vi "ParseAgentMessageChunk.vi"(8 "Error In":errorcluster, 9 "AgentMessage":T5, 10 "SessionId":string, 11 "LiteAgent In":T1) -> (0 "Error Out":errorcluster, 1 "Completions":T3, 2 "Part":T2, 3 "LiteAgent Out":T1, 5 "Common":T4)   [LabVIEW 2017]
uses:
  C:/Users/Jan/Projects/LiteAgentSDK-LabVIEW/Source/Bin/LiteAgentSDK.LabVIEW.dll
  Bin/LiteAgentSDK.LabVIEW.dll
  <vilib>/LVH/i3 JSON/i3-json.lvlib
  <vilib>/addons/Tools/Unicode/UTF8 Tools.lvlib
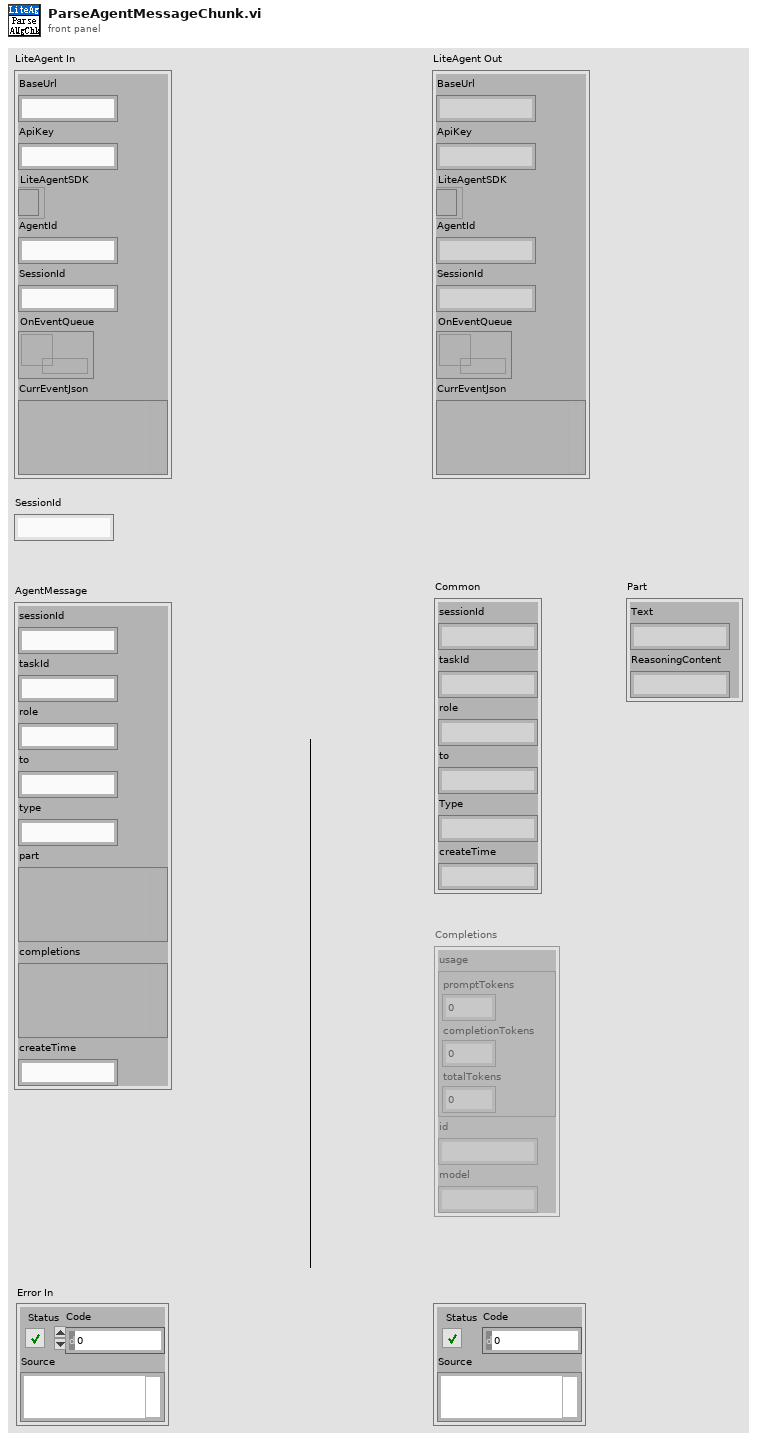
[diagram p1: front panel]
types:
  T1 = cluster{"BaseUrl":string, "ApiKey":string, "LiteAgentSDK":refnum<k24>, "AgentId":string, "SessionId":string, "OnEventQueue":refnum<queue>, "CurrEventJson":variant}
  T2 = cluster{"Text":string, "ReasoningContent":string}
  T3 = cluster{"usage":cluster{"promptTokens":i32, "completionTokens":i32, "totalTokens":i32}, "id":string, "model":string}
  T4 = cluster{"sessionId":string, "taskId":string, "role":string, "to":string, "Type":string, "createTime":string}
  T5 = cluster{"sessionId":string, "taskId":string, "role":string, "to":string, "type":string, "part":variant, "completions":variant, "createTime":string}
  T6 = enum8{"Enabled", "Disabled", "Disabled and Grayed Out"}
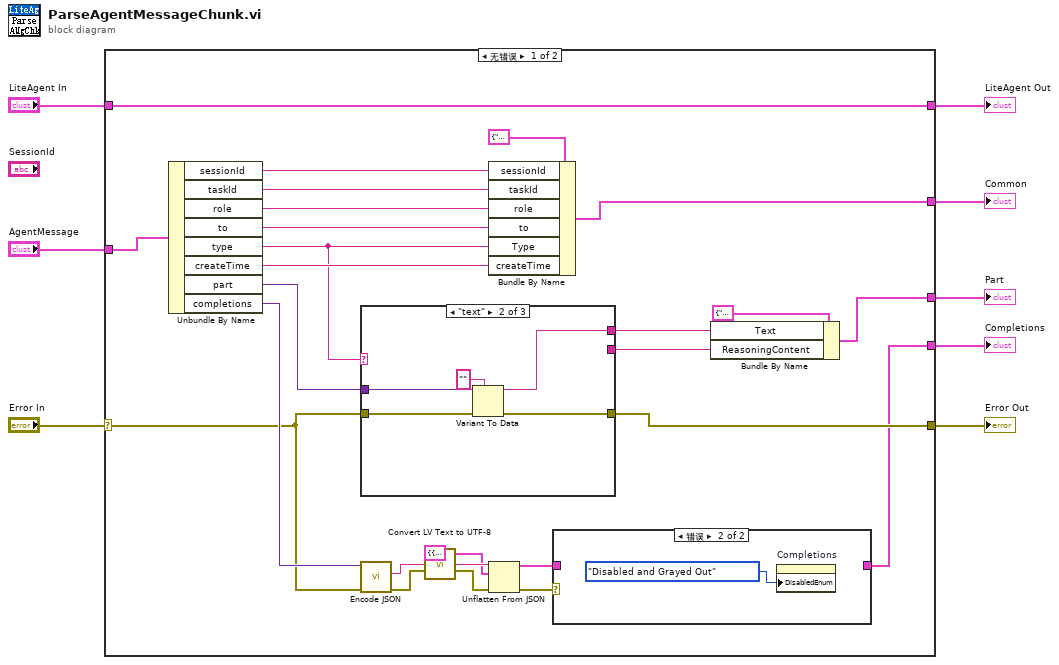
[diagram p0: block diagram]
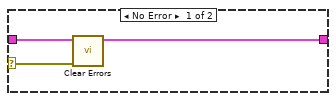
[diagram p2: hidden frame]
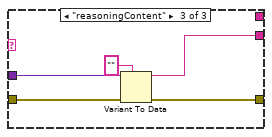
[diagram p4: hidden frame]
diagram:
  n1 = case shown="无错误" "Error In" {
    selector: "Error In" -> [w12 w50]
    tunnel: [w27 w50] -> w7
    tunnel: "AgentMessage" -> [w34 _]
    tunnel: [w29 _] -> w4
    tunnel: [w24 _] -> w1
    tunnel: [w23 _] -> w5
    tunnel: "LiteAgent In" -> [w19 w49]
    tunnel: [w19 w49] -> w2
    frame No Error {
      n2 = Unbundle By Name(w34) -> ("sessionId"=w33:string, "taskId"=w32:string, "role"=w31:string, "to"=w30:string, "type"=w20:string, "createTime"=w21:string, "part"=w28:variant, "completions"=w13:variant)
      n3 = case shown="\"text\"" w20 {
        tunnel: w28 -> [_ w43 w45]
        tunnel: w12 -> [w38 w42 w47]
        tunnel: [w38 w41 w46] -> w27
        tunnel: [_ w39 _] -> w26
        tunnel: [_ _ w44] -> w25
        frame "", Default {
        }
        frame "text" {
          n4 = Variant To Data(error in=w42, type="", Variant=w43) -> (data=w39:string, error out=w41:errorcluster)
        }
        frame "reasoningContent" {
          n5 = Variant To Data(error in=w47, type="", Variant=w45) -> (data=w44:string, error out=w46:errorcluster)
        }
      }
      n6 = call <vilib>:"Encode JSON.vi"("error in (no error)"=w12, "JSON Tree"=w13) -> ("error out"=w14:errorcluster, "String"=w17:string)  [unwired: 4 in]
      n7 = call <vilib>:"Convert LV Text to UTF-8.vi"("LV Text"=w17, "error in"=w14) -> ("UTF-8 Text"=w16:string, "error out"=w15:errorcluster)  [unwired: 12 in]
      n8 = Bundle By Name(cluster=T4 {"sessionId"="", "taskId"="", "role"="", "to"="", "Type"="", "createTime"=""} ("Common"), "sessionId"=w33, "taskId"=w32, "role"=w31, "to"=w30, "Type"=w20, "createTime"=w21) -> (w29:T4)
      n9 = Unflatten From JSON(JSON string=w16, type and defaults=T3 {"usage"={"promptTokens"=0, "completionTokens"=0, "totalTokens"=0}, "id"="", "model"=""} ("Completions"), error in (no error)=w15) -> (value=w9:T3, error out=w11:errorcluster)  [unwired: 4 in]
      n10 = case shown="错误" w11 {
        selector: w11 -> [w35 _]
        tunnel: w9 -> [w36 _]
        tunnel: [w36 _] -> w23
        frame No Error {
          n11 = call <vilib>:"Clear Errors.vi"("error in (no error)"=w35) -> ()  [unwired: 5 in, 2 out]
        }
        frame Error {
          n12 = property on="Completions" class="Clust (严格)"("DisabledEnum"=T6."Disabled and Grayed Out" ("禁用")) -> ()  [unwired: 2 in, 2 out]
        }
      }
      n13 = Bundle By Name(cluster=T2 {"Text"="", "ReasoningContent"=""} ("Part"), "Text"=w26, "ReasoningContent"=w25) -> (w24:T2)
    }
    frame Error {
    }
  }
  "Error Out" <- w7
  "Common" <- w4
  "Completions" <- w5
  "Part" <- w1
  "LiteAgent Out" <- w2
